vi "Localization - Apply.vi"(8 "Error In":errorcluster, 9 "Localization to Apply":i32, 10 "Control Class Array":refnum<class "Control Info.lvclass">[](array[class]), 11 "VI Reference":refnum<vi>) -> (0 "Error Out":errorcluster)   [LabVIEW 2017, in "Localization.lvlib"]
doc: "Applies the indicated column from the Localization for each control in the input array. VI Reference is used to defer front panel updates until all of the localizations have been applied.\n\n01/2020 Choose Movement Consulting, LLC"
uses:
  Localization.lvlib
  Control Info/Control Info.lvclass
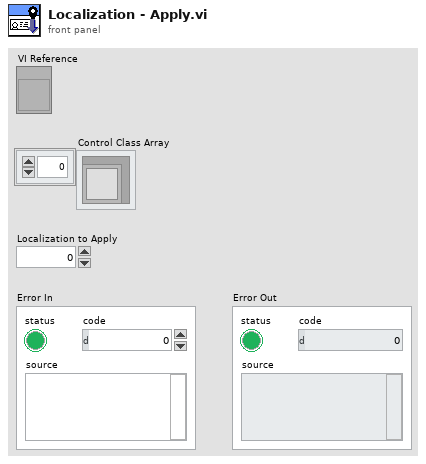
[diagram p1: front panel]
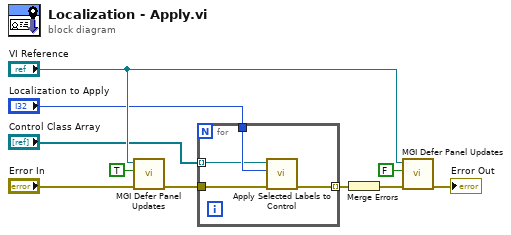
[diagram p0: block diagram]
diagram:
  n1 = call <userlib>:"MGI Defer Panel Updates.vi"("Error In"="Error In", "Defer Updates?"=TRUE, "VI Reference (Caller)"="VI Reference") -> ("Error Out"=w9:errorcluster)  [unwired: 8 in]
  n2 = for {
    tunnel: [w14] -> w7 mode=indexing
    tunnel: "Localization to Apply" -> [w13]
    tunnel: "Control Class Array" -> [w12] mode=indexing
    tunnel: w9 -> [w11]
    n3 = call-dynamic "Apply Selected Labels to Control.vi"("error in (no error)"=w11, "Alternate Text Select (0)"=w13, "Control Info in"=w12) -> ("error out"=w14:errorcluster)  [unwired: 7 in, 1 out]
  }
  n4 = Merge Errors(w7) -> (w5:errorcluster)
  n5 = call <userlib>:"MGI Defer Panel Updates.vi"("Error In"=w5, "Defer Updates?"=FALSE, "VI Reference (Caller)"="VI Reference") -> ("Error Out"=→"Error Out":errorcluster)  [unwired: 8 in]
